vi "Is potential destination.vi"(8 "error in (no error)":errorcluster, 10 "Square":T1={"File"=enum."d", "Rank"=enum."4"}, 11 "Position in":refnum<class "Position.lvclass">) -> (0 "error out":errorcluster, 2 "Potential destination":bool, 3 "Position out":refnum<class "Position.lvclass">)   [LabVIEW 2016, in "Chesslib.lvlib" / "Position.lvclass"]
uses:
  Position.lvclass
  typedef/Square.ctl
  typedef/File.ctl
  typedef/Rank.ctl
  Position.lvclass/Position.ctl
  Pieces/Piece/Piece.lvclass/Piece.ctl
  Board/Board.lvclass
  Pieces/Piece/Piece.lvclass
  Chesslib.lvlib
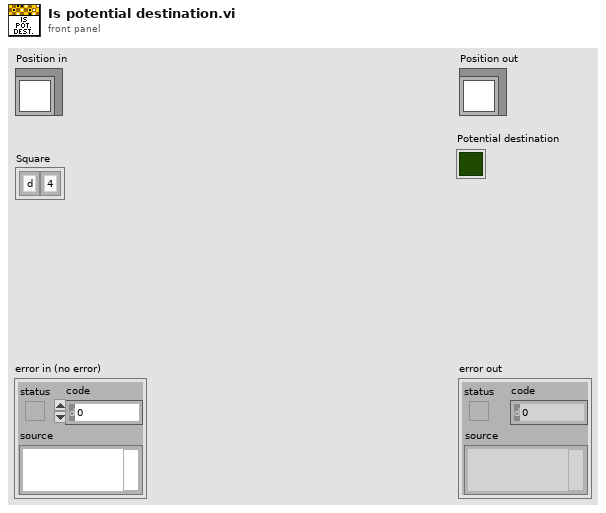
[diagram p1: front panel]
types:
  T1 = typedef "Chesslib.lvlib/Square.ctl" = cluster{"File":T2, "Rank":T3}
  T2 = typedef "Chesslib.lvlib/File.ctl" = enum8{"a", "b", "c", "d", "e", "f", "g", "h"}
  T3 = typedef "Chesslib.lvlib/Rank.ctl" = enum8{"1", "2", "3", "4", "5", "6", "7", "8"}
  T4 = typedef "Chesslib.lvlib/Color.ctl" = enum16{"Light", "Dark"}
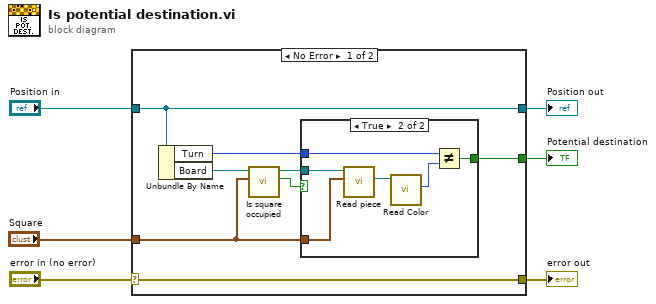
[diagram p0: block diagram]
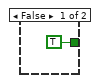
[diagram p2: hidden frame]
diagram:
  n1 = case shown="No Error" "error in (no error)" {
    selector: "error in (no error)" -> [w7 w23]
    tunnel: [w7 w23] -> w5
    tunnel: [w14 w22] -> w3
    tunnel: "Position in" -> [w14 w22]
    tunnel: "Square" -> [w10 _]
    tunnel: [w8 _] -> w1
    frame No Error {
      n2 = Unbundle By Name(w14) -> ("Turn"=w9:T4, "Board"=w13:refnum<class "Board.lvclass">)
      n3 = call "Is square occupied.vi"("Square"=w10, "Board in"=w13) -> ("Occupied"=w12:bool, "Board out"=w11:refnum<class "Board.lvclass">)  [unwired: 7 in, 1 out]
      n4 = case shown="True" w12 {
        tunnel: w11 -> [_ w21]
        tunnel: w10 -> [_ w20]
        tunnel: w9 -> [_ w18]
        tunnel: [TRUE w16] -> w8
        frame False {
        }
        frame True {
          n5 = call "Read piece.vi"("Square"=w20, "Board in"=w21) -> ("Piece"=w19:refnum<class "Piece.lvclass">)  [unwired: 7 in, 2 out]
          n6 = call "Read Color.vi"("Piece in"=w19) -> ("Color"=w17:T4)  [unwired: 10 in]
          n7 = Not Equal?(x=w18, y=w17) -> (x != y?=w16:bool)
        }
      }
    }
    frame Error {
    }
  }
  "error out" <- w5
  "Position out" <- w3
  "Potential destination" <- w1
